vi "Temperature Limit.vi"() -> ()   [LabVIEW 2012]
doc: "该VI可仿真温度采集，绘制温度图形，并通知用户温度是否超出范围。"
panel:
  in  "开始":bool
  in  "△t(ms)":i32(slide)=400 scale=50.0..500.0
  in  "停止":bool
  in  "上限":dbl=28.0 format="%.2f"
  out "温度":cluster{"Temperature":dbl, "High Limit":dbl}(graph)={"Temperature"=85.88749999999999, "High Limit"=80.0}
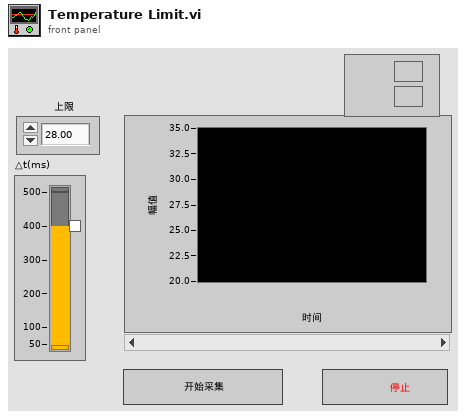
[diagram p1: front panel]
types:
  T1 = enum16{"Always On", "Always Off", "Off While Running"}
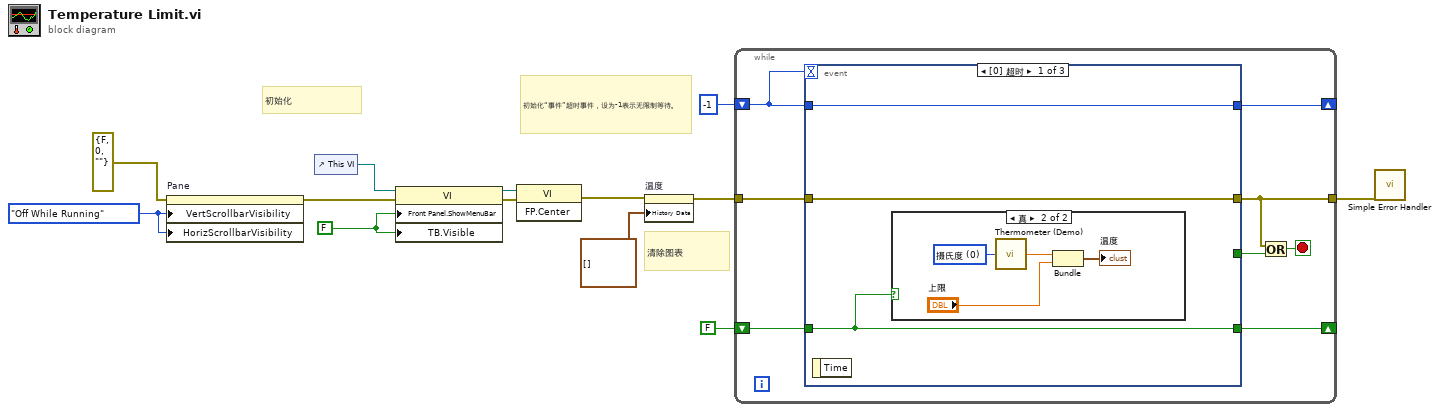
[diagram p0: block diagram]
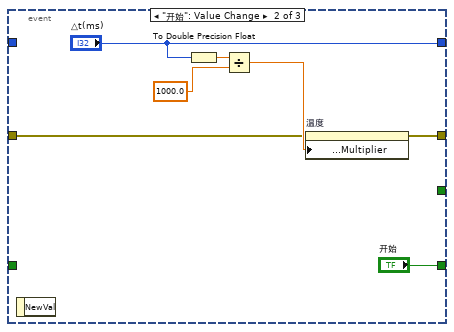
[diagram p3: hidden frame]
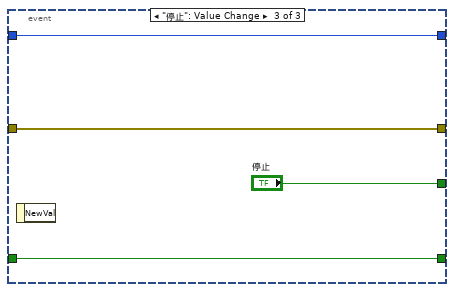
[diagram p4: hidden frame]
diagram:
  w3 = T1."Off While Running" ("水平滚动条可见")
  w8 = FALSE
  # "清除图表"
  # "初始化“事件”超时事件，设为-1表示无限制等待。"
  # "初始化"
  n1 = property on="Pane" class="Pane"(error in=cluster{"状态":bool, "代码":i32, "源":string} {"状态"=FALSE, "代码"=0, "源"=""} ("错误输入（无错误）"), "VertScrollbarVisibility"=w3, "HorizScrollbarVisibility"=w3) -> (error out=w4:errorcluster)  [unwired: 1 in, 1 out]
  n2 = control-ref of="This VI"() -> (w5:refnum<vi>)
  n3 = property on="属性节点" class="VI"(reference=w5, error in=w4, "Front Panel.ShowMenuBar"=w8, "TB.Visible"=w8) -> (reference out=w7:refnum<vi>, error out=w6:errorcluster)
  n4 = invoke on="调用节点" class="VI" method="FP.Center"(reference=w7, error in=w6) -> (error out=w2:errorcluster)  [unwired: 1 in, 2 out]
  n5 = property on="温度" class="WFChart (严格)"(error in=w2, "History Data"=cluster{"温度":dbl, "高限制":dbl}[] [] ("历史数据")) -> (error out=w12:errorcluster)  [unwired: 1 in, 1 out]
  n6 = while {
    tunnel: w12 -> [w21]
    tunnel: [w19] -> w10
    shift-right: [w17] -> _
    shift-left: FALSE ("开始") -> [w16]
    shift-right: [w15] -> _
    shift-left: -1 ("△t(ms)") -> [w14]
    stop <- w20 stop-if-true
    n7 = event shown="[0] 超时" {
      selector: _ -> [_ _ _]
      dyn-events: _ -> [_ _ _]
      timeout: w14 -> [_ _ _]
      tunnel: [_ _ "停止"] -> w18
      tunnel: w21 -> [w24 w29 w38]
      tunnel: [w24 w35 w38] -> w19
      tunnel: [w22 "开始" w37] -> w17
      tunnel: w16 -> [w22 _ w37]
      tunnel: [w23 "△t(ms)" w36] -> w15
      tunnel: w14 -> [w23 _ w36]
      event Timeout {
        n8 = event-data ("事件数据节点")() -> ()  [unwired: 1 in, 1 out]
        n9 = case shown="真" w22 {
          frame False {
          }
          frame True {
            w25 = u16 0 items=["摄氏度", "华氏度"] ("单位（0：摄氏度）")
            n10 = call "Thermometer (Demo).vi"("单位（0：摄氏度）"=w25) -> ("温度值"=w26:dbl)
            n11 = Bundle ("捆绑")("温度值"=w26, "上限"="上限") -> (→"温度":cluster{"温度值":dbl, "上限":dbl})  [unwired: 1 in]
          }
        }
      }
      event "开始": Value Change {
        n12 = event-data ("事件数据节点")() -> ()  [unwired: 1 in, 1 out]
        n13 = To Double Precision Float ("转换为双精度浮点数")(number="△t(ms)") -> (double precision float=w34:dbl)
        n14 = Divide ("除")(x=w34, y=1000.0) -> (x/y=w32:dbl)
        n15 = property on="温度" class="WFChart (严格)"(error in=w29, "X Scale.Offset and Multiplier:Multiplier"=w32) -> (error out=w35:errorcluster)  [unwired: 1 in, 1 out]
      }
      event "停止": Value Change {
        n16 = event-data ("事件数据节点")() -> ()  [unwired: 1 in, 1 out]
      }
    }
    n17 = Or ("或")(x=w19, y=w18) -> (x .or. y?=w20:bool)
  }
  n18 = call <vilib>:"Simple Error Handler.vi"("error in (no error)"=w10) -> ()  [unwired: 4 in, 5 out]
